vi "Init(Camera).vi"(8 "error in (no error)":errorcluster, 10 "Camera_Settings_Ref":refnum<vi>, 11 "Session in":T1) -> (0 "error out":errorcluster, 3 "Session out":T1)   [LabVIEW 2020]
uses:
  <vilib>/userDefined/High Color/IMAQdx.ctl
  Controls/Camera_Settings.ctl
  <resource>/objmgr/imaqdx.rc
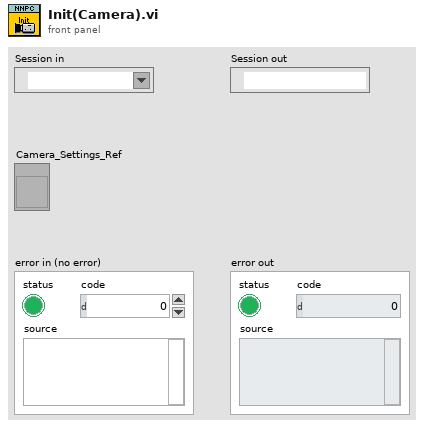
[diagram p1: front panel]
types:
  T1 = typedef "IMAQdx.ctl" = refnum<k21>
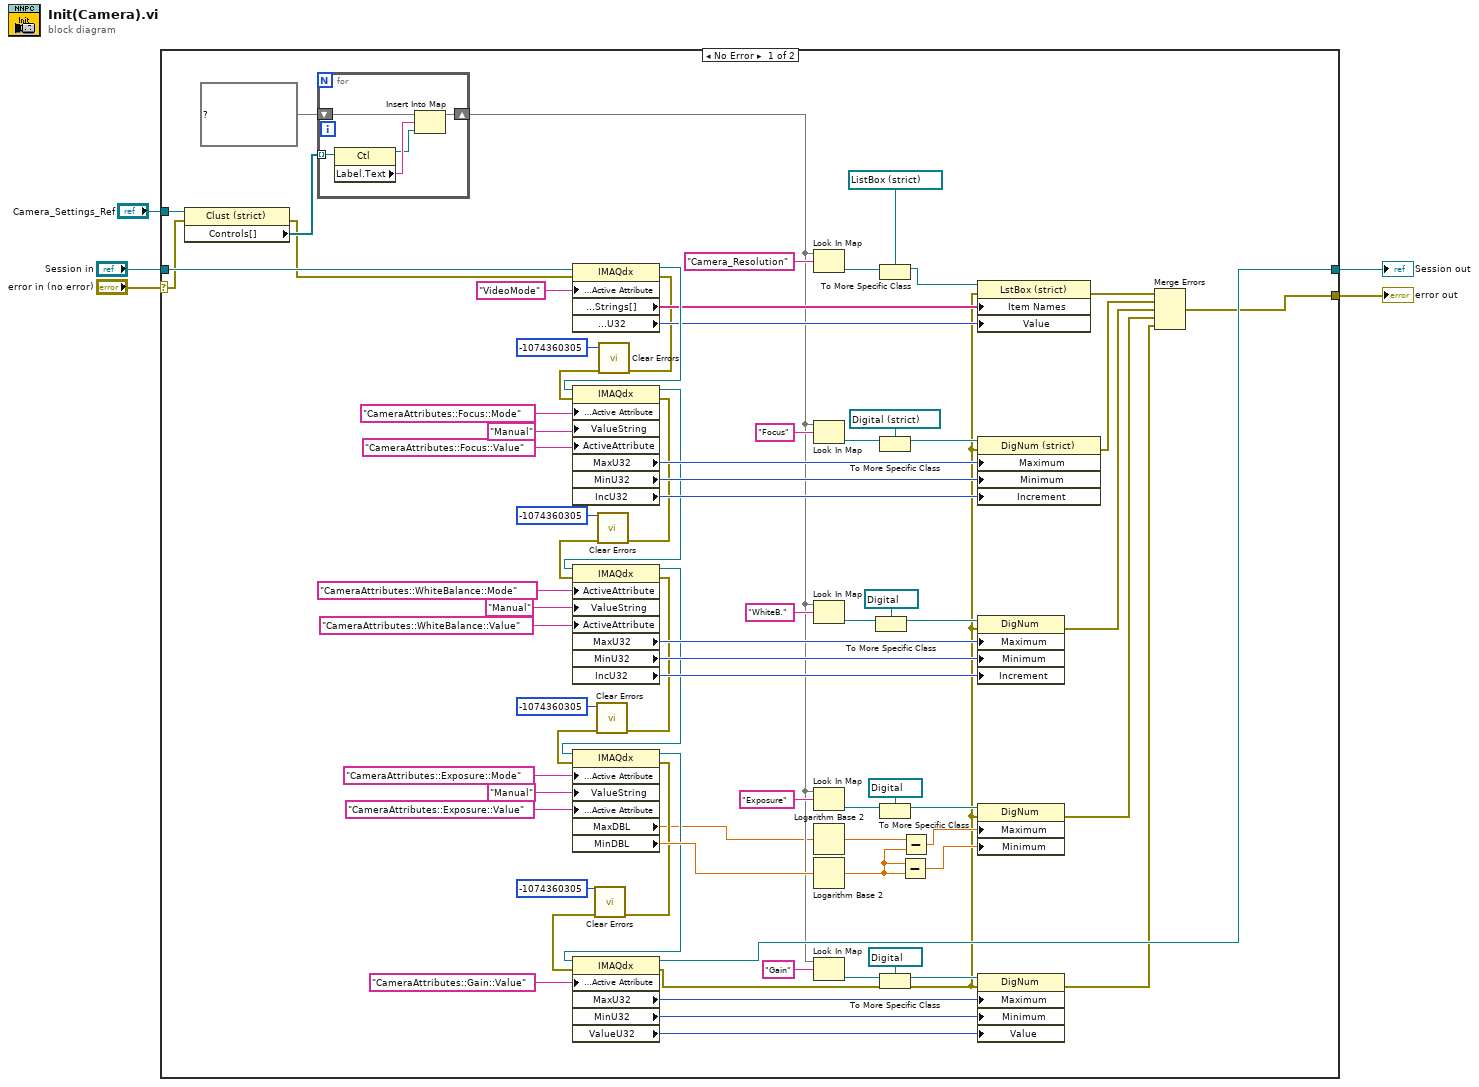
[diagram p0: block diagram]
diagram:
  n1 = case shown="No Error" "error in (no error)" {
    selector: "error in (no error)" -> [w39 w91]
    tunnel: [w73 w90] -> w5
    tunnel: [w14 w91] -> w4
    tunnel: "Camera_Settings_Ref" -> [w63 _]
    tunnel: "Session in" -> [w40 w90]
    frame No Error {
      n2 = property class="Clust (strict)"(reference=w63, error in=w39) -> (error out=w38:errorcluster, "Controls[]"=w62:refnum<vi>[])  [unwired: 1 out]
      n3 = for {
        tunnel: w62 -> [w89] mode=indexing
        shift-right: [w85] -> w26
        shift-left: map{string, refnum<vi>} {} ("map") -> [w88]
        n4 = property class="Ctl"(reference=w89) -> (reference out=w86:refnum<vi>, "Label.Text"=w87:string)  [unwired: 1 in, 1 out]
        n5 = Insert Into Map(map in=w88, key=w87, value=w86) -> (map out=w85:map{string, refnum<vi>})  [unwired: 2 out]
      }
      n6 = property class="IMAQdx"(reference=w40, error in=w38, "Camera Attributes:Active Attribute"="VideoMode" ("ActiveAttribute")) -> (reference out=w67:T1, error out=w24:errorcluster, "Camera Attributes:Enum:Strings[]"=w65:string[], "Camera Attributes:Value:U32"=w66:u32)
      n7 = call <vilib>:"Clear Errors.vi"("error in (no error)"=w24, "specific error code to clear (0: all)"=-1074360305) -> ("error out"=w13:errorcluster)  [unwired: 4 in, 1 out]
      n8 = property class="IMAQdx"(reference=w67, error in=w13, "Camera Attributes:Active Attribute"="CameraAttributes::Focus::Mode" ("ActiveAttribute"), "ValueString"="Manual", "ActiveAttribute"="CameraAttributes::Focus::Value") -> (reference out=w46:T1, error out=w25:errorcluster, "MaxU32"=w82:u32, "MinU32"=w83:u32, "IncU32"=w84:u32)
      n9 = call <vilib>:"Clear Errors.vi"("error in (no error)"=w25, "specific error code to clear (0: all)"=-1074360305) -> ("error out"=w12:errorcluster)  [unwired: 4 in, 1 out]
      n10 = property class="IMAQdx"(reference=w46, error in=w12, "ActiveAttribute"="CameraAttributes::WhiteBalance::Mode", "ValueString"="Manual", "ActiveAttribute"="CameraAttributes::WhiteBalance::Value") -> (reference out=w45:T1, error out=w23:errorcluster, "MaxU32"=w50:u32, "MinU32"=w51:u32, "IncU32"=w52:u32)
      n11 = call <vilib>:"Clear Errors.vi"("error in (no error)"=w23, "specific error code to clear (0: all)"=-1074360305) -> ("error out"=w11:errorcluster)  [unwired: 4 in, 1 out]
      n12 = property class="IMAQdx"(reference=w45, error in=w11, "Camera Attributes:Active Attribute"="CameraAttributes::Exposure::Mode" ("ActiveAttribute"), "ValueString"="Manual", "Camera Attributes:Active Attribute"="CameraAttributes::Exposure::Value" ("ActiveAttribute")) -> (reference out=w72:T1, error out=w22:errorcluster, "MaxDBL"=w21:dbl, "MinDBL"=w78:dbl)
      n13 = call <vilib>:"Clear Errors.vi"("error in (no error)"=w22, "specific error code to clear (0: all)"=-1074360305) -> ("error out"=w10:errorcluster)  [unwired: 4 in, 1 out]
      n14 = property class="IMAQdx"(reference=w72, error in=w10, "Camera Attributes:Active Attribute"="CameraAttributes::Gain::Value" ("ActiveAttribute")) -> (reference out=w73:T1, error out=w18:errorcluster, "MaxU32"=w71:u32, "MinU32"=w70:u32, "ValueU32"=w69:u32)
      n15 = Look In Map(map=w26, key="Camera_Resolution") -> (value=w35:refnum<vi>)  [unwired: 1 in, 1 out]
      n16 = Look In Map(map=w26, key="Focus") -> (value=w30:refnum<vi>)  [unwired: 1 in, 1 out]
      n17 = Look In Map(map=w26, key="WhiteB.") -> (value=w29:refnum<vi>)  [unwired: 1 in, 1 out]
      n18 = Look In Map(map=w26, key="Exposure") -> (value=w28:refnum<vi>)  [unwired: 1 in, 1 out]
      n19 = Logarithm Base 2(1:w21) -> (0:w76:dbl)
      n20 = Logarithm Base 2(1:w78) -> (0:w77:dbl)
      n21 = Look In Map(map=w26, key="Gain") -> (value=w27:refnum<vi>)  [unwired: 1 in, 1 out]
      n22 = To More Specific Class(target class=refnum<vi> refnum ("DigNum Refnum"), reference=w29) -> (specific class reference=w56:refnum<vi>)  [unwired: 1 in, 1 out]
      n23 = To More Specific Class(target class=refnum<vi> refnum ("ListBox in"), reference=w35) -> (specific class reference=w54:refnum<vi>)  [unwired: 1 in, 1 out]
      n24 = To More Specific Class(target class=refnum<vi> refnum ("DigNum Refnum 5"), reference=w30) -> (specific class reference=w53:refnum<vi>)  [unwired: 1 in, 1 out]
      n25 = To More Specific Class(target class=refnum<vi> refnum ("DigNum Refnum"), reference=w28) -> (specific class reference=w58:refnum<vi>)  [unwired: 1 in, 1 out]
      n26 = To More Specific Class(target class=refnum<vi> refnum ("DigNum Refnum"), reference=w27) -> (specific class reference=w57:refnum<vi>)  [unwired: 1 in, 1 out]
      n27 = Subtract(x=w77, y=w77) -> (x-y=w80:dbl)
      n28 = Subtract(x=w76, y=w77) -> (x-y=w79:dbl)
      n29 = property on="Property Node" class="LstBox (strict)"(reference=w54, error in=w18, "Item Names"=w65, "Value"=w66) -> (error out=w20:errorcluster)  [unwired: 1 out]
      n30 = property on="Property Node" class="DigNum (strict)"(reference=w53, error in=w18, "Maximum"=w82, "Minimum"=w83, "Increment"=w84) -> (error out=w19:errorcluster)  [unwired: 1 out]
      n31 = property on="Property Node" class="DigNum"(reference=w56, error in=w18, "Maximum"=w50, "Minimum"=w51, "Increment"=w52) -> (error out=w17:errorcluster)  [unwired: 1 out]
      n32 = property on="Property Node" class="DigNum"(reference=w58, error in=w18, "Maximum"=w79, "Minimum"=w80) -> (error out=w16:errorcluster)  [unwired: 1 out]
      n33 = property on="Property Node" class="DigNum"(reference=w57, error in=w18, "Maximum"=w71, "Minimum"=w70, "Value"=w69) -> (error out=w15:errorcluster)  [unwired: 1 out]
      n34 = Merge Errors(w20, w19, w17, w16, w15) -> (w14:errorcluster)
    }
    frame Error {
    }
  }
  "Session out" <- w5
  "error out" <- w4
